vi "BPSK_rx.vi"() -> ()   [LabVIEW 2022 SP3]
uses:
  <vilib>/measure/NI_MAPro.lvlib
  <vilib>/measure/madcrms.llb/Basic Averaged DC-RMS for N Chan.vi
  <vilib>/Analysis/NI_AALPro.lvlib
  <instrlib>/niUSRP/niUSRP Fetch Rx Data (CDB).vi
panel:
  out "rx  signal":dbl[](graph)
  in  "stop":bool
  out "Constellation":cluster{i32[], i32[]}(graph)
  out "Array 1":i32[](array[numeric])
  out "Array 2":i32[](array[numeric])
  out "BER":dbl
  out "sum":dbl
  out "output Array 2":dbl[](array[numeric])
  in  "for loop":i32
  out "output array":dbl[](array[numeric])
  out "Output 2":dbl
  in  "active antenna":string
  in  "gain":dbl format="%#_6f"
  in  "carrier frequency":dbl=100000.0 format="%#_6p"
  in  "IQ rate":dbl=100000.0 format="%#_6p"
  in  "device names":refnum<k15>
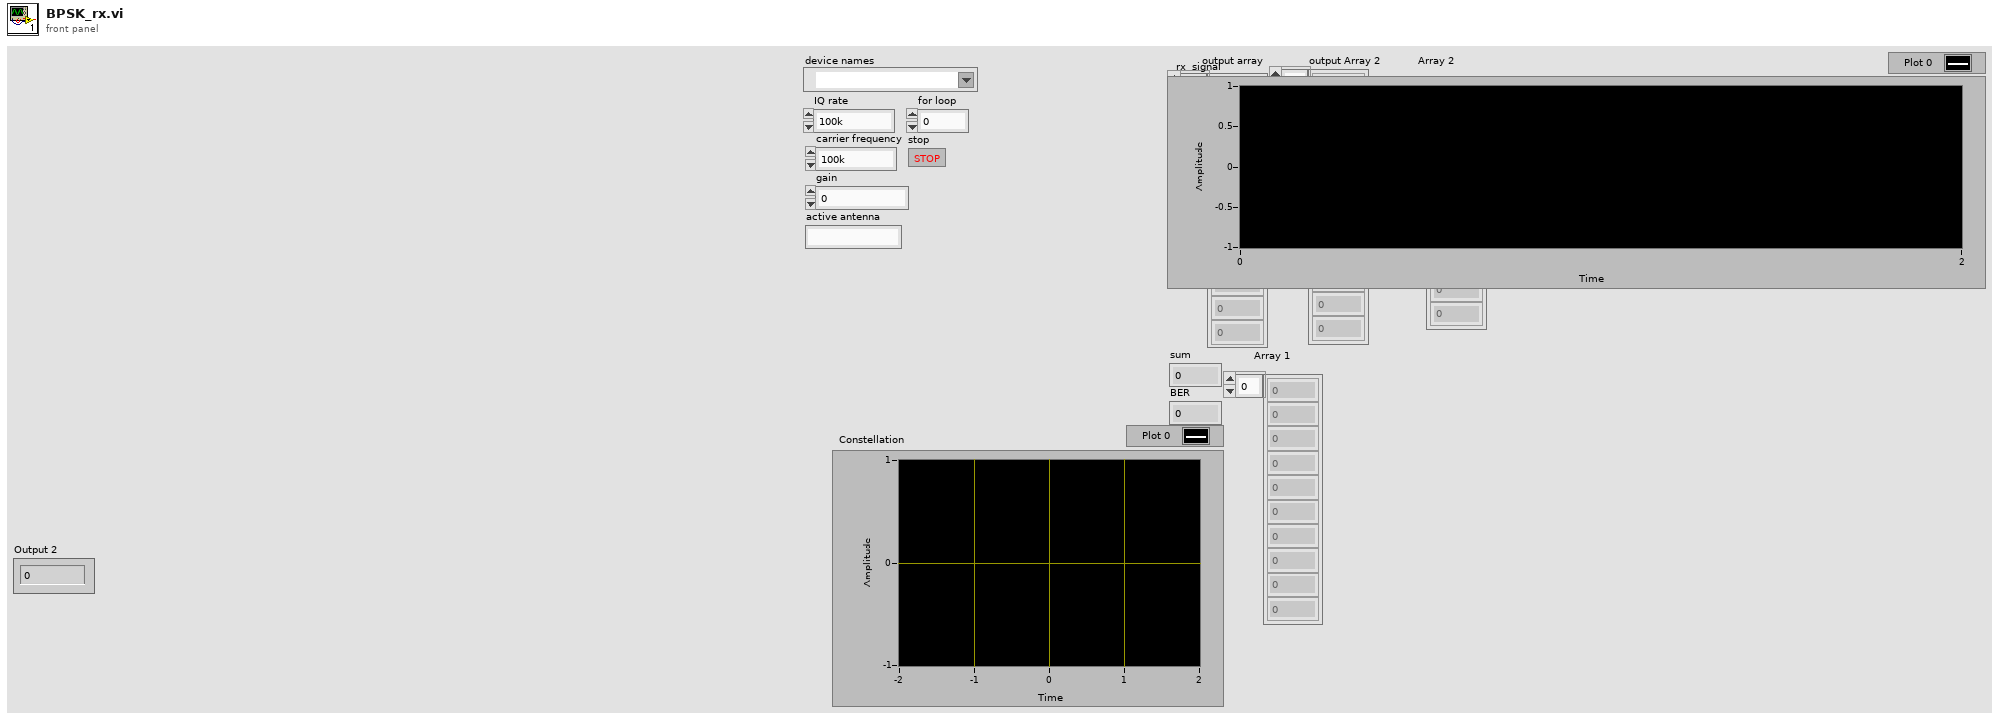
[diagram p1: front panel]
types:
  T1 = enum16{"sine", "cosine", "triangle", "square", "sawtooth", "increasing ramp", "decreasing ramp"}
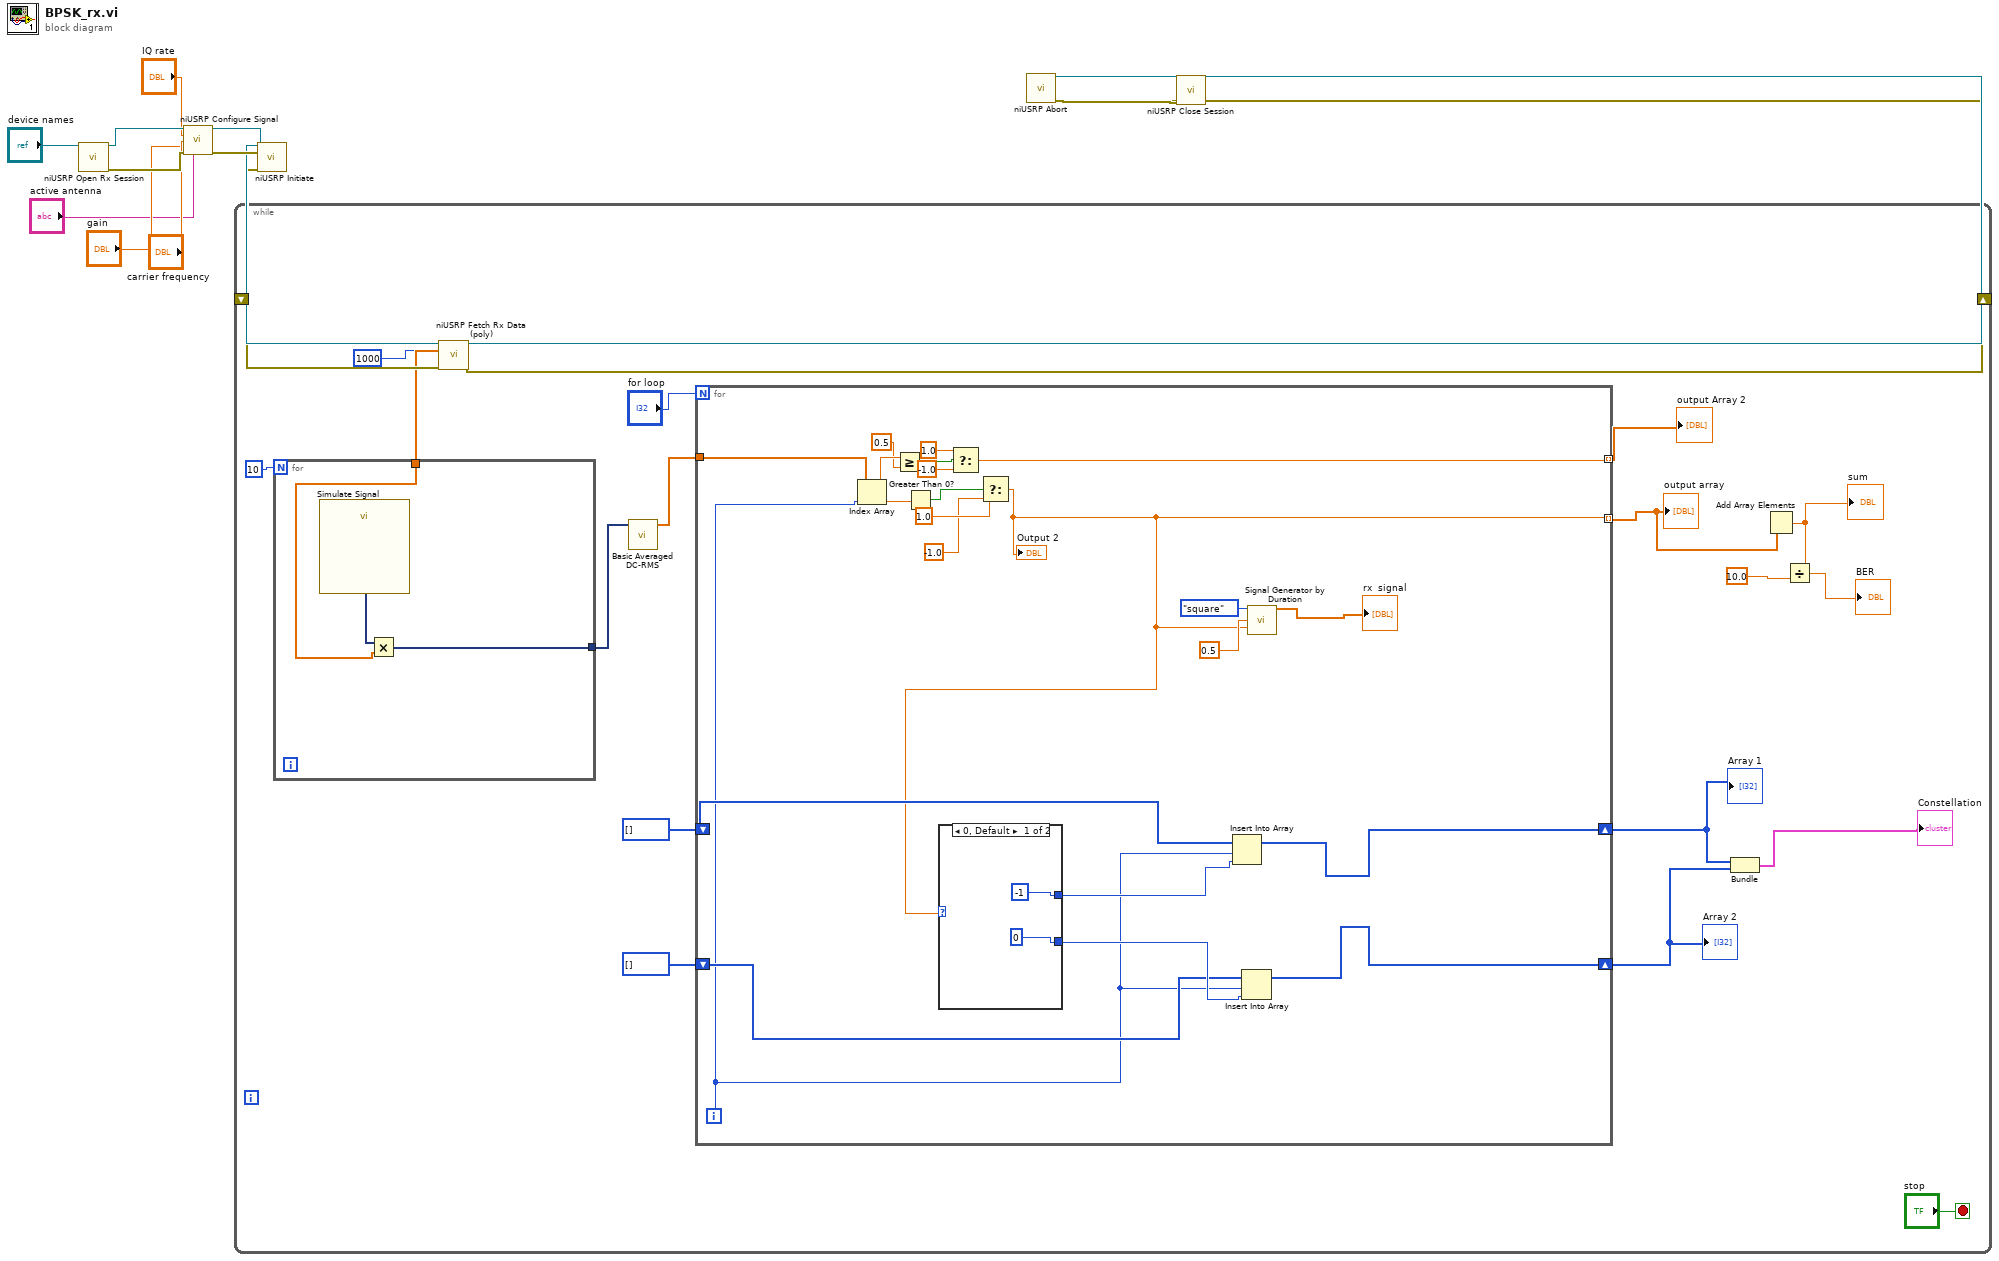
[diagram p0: block diagram]
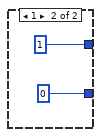
[diagram p2: hidden frame]
diagram:
  n1 = call <instrlib>:"niUSRP Open Rx Session.vi"("device names"="device names") -> ("session handle out"=w13:refnum<k15>, "error out"=w12:errorcluster)  [unwired: 13 in]
  n2 = call <instrlib>:"niUSRP Configure Signal.vi"("session handle"=w13, "IQ rate"="IQ rate", "carrier frequency"="carrier frequency", "gain"="gain", "error in (no error)"=w12, "active antenna"="active antenna") -> ("session handle out"=w15:refnum<k15>, "error out"=w14:errorcluster)  [unwired: 5 in, 3 out]
  n3 = call <instrlib>:"niUSRP Initiate.vi"("session handle"=w15, "error in (no error)"=w14) -> ("session handle out"=w4:refnum<k15>, "error out"=w3:errorcluster)  [unwired: 12 in]
  n4 = while {
    shift-right: [w32] -> w2
    shift-left: w4 -> [w34]
    shift-right: [w30] -> w1
    shift-left: w3 -> [w33]
    stop <- "stop" stop-if-true
    n5 = call-poly <instrlib>:"niUSRP Fetch Rx Data (poly).vi"("session handle"=w34, "number of samples"=i64 1000, "error in (no error)"=w33) -> ("session handle out"=w32:refnum<k15>, "data"=w31:cdb[], "error out"=w30:errorcluster)  [unwired: 9 in, 1 out]
    n6 = for {
      N: 10 -> [_]
      tunnel: [w63] -> w27
      tunnel: w31 -> [w62]
      n7 = call "Simulate Signal"() -> ("Sine"=w64:dynamicdata)  [unwired: 14 in, 1 out]
      n8 = Multiply(x=w64, y=w62) -> (x*y=w63:dynamicdata[])
    }
    n9 = call-poly <vilib>:"Basic Averaged DC-RMS.vi"("signals in"=w27) -> ("DC values"=w28:dbl[])  [unwired: 7 in, 3 out]
    n10 = for {
      N: "for loop" -> [_]
      tunnel: w28 -> [w54]
      tunnel: [w38] -> w26 mode=indexing
      tunnel: [w48] -> w16 mode=indexing
      shift-right: [w42] -> w19
      shift-left: i32[] [] -> [w44]
      shift-right: [w41] -> w18
      shift-left: i32[] [] -> [w45]
      i -> [w43]
      n11 = Index Array(array=w54, index=w43) -> (element=w53:dbl)
      n12 = Greater Or Equal?(x=w53, y=0.5) -> (x >= y?=w51:bool)
      n13 = Greater Than 0?(x=w53) -> (x > 0?=w57:bool)
      n14 = Select(t=1.0, s=w51, f=-1.0) -> (s? t:f=w48:dbl)
      n15 = Select(t=1.0, s=w57, f=-1.0) -> (s? t:f=w38:dbl)
      "Output 2" <- w38
      n16 = case shown="0, Default" w38 {
        tunnel: [-1 1] -> w47
        tunnel: [0 0] -> w46
        frame 0, Default {
        }
        frame 1 {
        }
      }
      n17 = Insert Into Array(array=w44, index=w43, new element=w47) -> (w42:i32[])
      n18 = Insert Into Array(array=w45, index=w43, new element=w46) -> (w41:i32[])
      n19 = call <vilib>:"Signal Generator by Duration.vi"("signal type"=T1."square", "frequency"=0.5, "amplitude"=w38) -> ("signal"=→"rx  signal":dbl[])  [unwired: 9 in, 3 out]
    }
    "output array" <- w26
    "output Array 2" <- w16
    "Array 2" <- w18
    "Array 1" <- w19
    n20 = Bundle(w19, w18) -> (→"Constellation":cluster{i32[], i32[]})  [unwired: 1 in]
    n21 = Add Array Elements(numeric array=w26) -> (sum=w25:dbl)
    "sum" <- w25
    n22 = Divide(x=w25, y=10.0) -> (x/y=→"BER":dbl)
  }
  n23 = call <instrlib>:"niUSRP Abort.vi"("session handle"=w2, "error in (no error)"=w1) -> ("session handle out"=w6:refnum<k15>, "error out"=w5:errorcluster)  [unwired: 12 in]
  n24 = call <instrlib>:"niUSRP Close Session.vi"("session handle"=w6, "error in (no error)"=w5) -> ()  [unwired: 13 in, 1 out]
